vi "FTW-Regex-Execute.vi"(0 "Regex":refnum<data-value>, 5 "Subject String":string, 7 "Starting Offset":i32, 11 "error in":errorcluster) -> (4 "Regex out":refnum<data-value>, 6 "Whole Match Begin":i32, 8 "Offset after Match":i32, 10 "Submatches":i32[](array[numeric]), 14 "Callouts":T1(array[cluster]), 15 "error out":errorcluster)   [LabVIEW 2015]
uses:
  core/FTW-Regex-Core-Structure.ctl
panel:
  # "Inputs"
  # "Outputs"
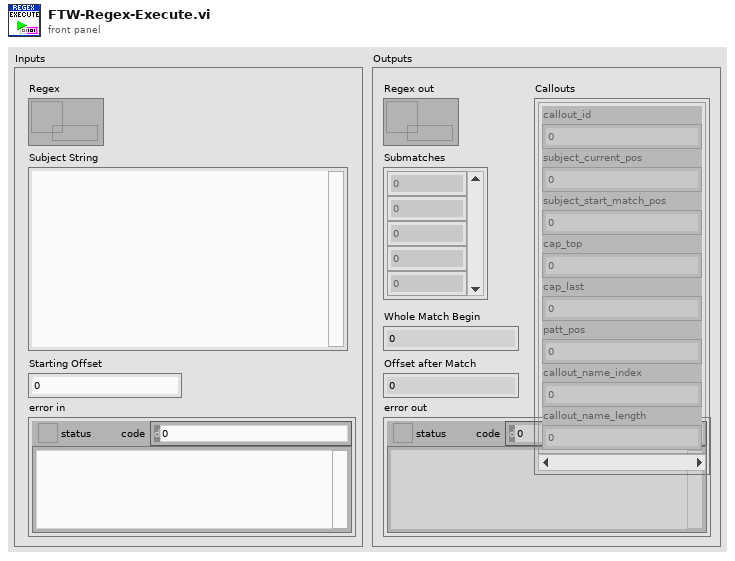
[diagram p1: front panel]
types:
  T1 = cluster{"callout_id":i32, "subject_current_pos":i32, "subject_start_match_pos":i32, "cap_top":i32, "cap_last":i32, "patt_pos":i32, "callout_name_index":i32, "callout_name_length":i32}[]
  T2 = typedef "FTW-Regex-Core-Structure.ctl" = cluster{"Compiled Regex":u64}
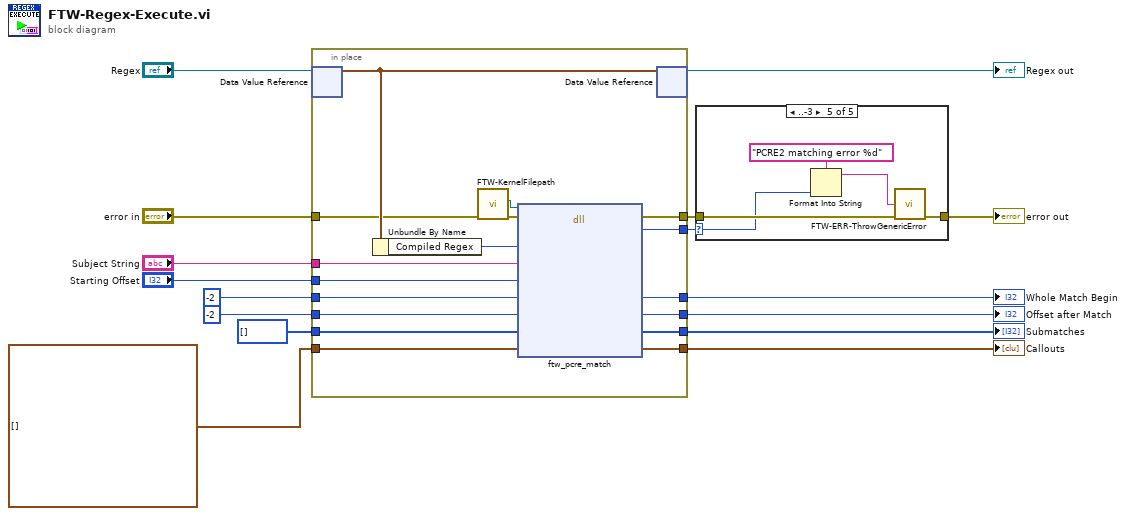
[diagram p0: block diagram]
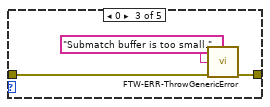
[diagram p4: hidden frame]
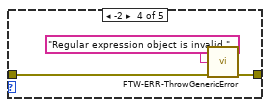
[diagram p5: hidden frame]
diagram:
  n1 = in-place {
    in-place-border: [w33] -> w9
    in-place-border: "error in" -> [w19]
    in-place-border: "Subject String" -> [w32]
    in-place-border: "Starting Offset" -> [w31]
    in-place-border: [w29] -> w13
    in-place-border: i32[] [] -> [w30]
    in-place-border: [w28] -> w12
    in-place-border: [w27] -> w3
    in-place-border: [w26] -> w11
    in-place-border: [w25] -> w8
    in-place-border: -2 -> [w24]
    in-place-border: -2 -> [w23]
    in-place-border: T1 [] ("Callouts") -> [w22]
    n2 = in-place-dvr #1("Regex") -> (w21:T2)  [unwired: 1 out]
    n3 = Unbundle By Name(w21) -> ("Compiled Regex"=w20:u64)
    n4 = call "FTW-KernelFilepath.vi"("error in"=w19) -> ("error out"=w18:errorcluster, "Library Filepath"=w17:path)  [unwired: 8 in, 1 out]
    n5 = dll-call lib="?" fn="ftw_pcre_match"(path in=w17, error in=w18, "Compiled Regex"=w20, "Subject String"=w32, "Starting Offset"=w31, "Match Begin"=w24, "Match End"=w23, "Submatch Buffer"=w30, "Callout Buffer"=w22) -> (error out=w33:errorcluster, "Return Value"=w26:i32, "Match Begin"=w25:i32, "Match End"=w29:i32, "Submatch Buffer"=w28:i32[], "Callout Buffer"=w27:T1)  [unwired: 4 in, 1 out]
    n6 = in-place-dvr #1(w21) -> (→"Regex out":refnum<data-value>)  [unwired: 1 out]
  }
  "Offset after Match" <- w13
  "Submatches" <- w12
  "Callouts" <- w3
  "Whole Match Begin" <- w8
  n7 = case shown="..-3" w11 {
    selector: w11 -> [_ _ _ _ w44]
    tunnel: [w34 w35 w37 w40 w45] -> w10
    tunnel: w9 -> [w34 w35 w38 w41 w46]
    frame 1.. {
      # "Match found and no error."
    }
    frame -1 {
      # "PCRE_ERROR_NOMATCH\nDon't treat this as an error!"
    }
    frame 0 {
      n8 = call "FTW-ERR-ThrowGenericError.vi"("Error Message"="Submatch buffer is too small.", "error in"=w38) -> ("error out"=w37:errorcluster)  [unwired: 13 in]
    }
    frame -2 {
      n9 = call "FTW-ERR-ThrowGenericError.vi"("Error Message"="Regular expression object is invalid.", "error in"=w41) -> ("error out"=w40:errorcluster)  [unwired: 13 in]
    }
    frame ..-3 {
      n10 = Format Into String(format string="PCRE2 matching error %d" ("Error Message"), w44) -> (resulting string=w43:string)  [unwired: 2 in, 1 out]
      n11 = call "FTW-ERR-ThrowGenericError.vi"("Error Message"=w43, "error in"=w46) -> ("error out"=w45:errorcluster)  [unwired: 13 in]
    }
  }
  "error out" <- w10
